vi "stopDAQ.vi"   [LabVIEW 2011]
uses:
  <vilib>/Utility/error.llb/DialogType.ctl
  GlobalDAQ.vi
types:
  T1 = typedef "DialogType.ctl" = u16
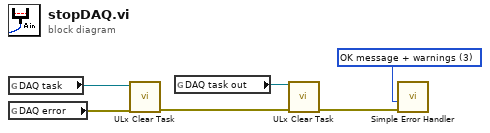
[diagram p0: block diagram]
diagram:
  w6 = T1 3 items=["no dialog", "OK message", "continue or stop message", "OK message + warnings", "continue/stop + warnings"] ("type of dialog (OK msg:1)")
  n1 = global read "GlobalDAQ.vi" "DAQ task"() -> (w5:refnum<k24>)
  n2 = global read "GlobalDAQ.vi" "DAQ error"() -> (w4:errorcluster)
  n3 = call <vilib>:"ULx Clear Task.vi"("task in"=w5, "error in"=w4) -> ("error out"=w2:errorcluster)  [unwired: 13 in]
  n4 = global read "GlobalDAQ.vi" "DAQ task out"() -> (w3:refnum<k24>)
  n5 = call <vilib>:"ULx Clear Task.vi"("task in"=w3, "error in"=w2) -> ("error out"=w1:errorcluster)  [unwired: 13 in]
  n6 = call <vilib>:"Simple Error Handler.vi"("type of dialog (OK msg:1)"=w6, "error in (no error)"=w1) -> ()  [unwired: 3 in, 5 out]
